vi "plot circles.vi"(2 "dL":dbl=0.5, 3 "Radius":dbl[](array[numeric])=[10.0, 5.0, 8.0, 1.0], 4 "Circle y":dbl[](array[numeric])=[0.0, 3.0, -7.0, -4.0], 5 "Circle x":dbl[](array[numeric])=[0.0, 4.0, -2.0, 2.0]) -> (0 "CY":dbl[](array[numeric]), 1 "CX":dbl[](array[numeric]))   [LabVIEW 2009]
panel:
  out "XY Graph":cluster{dbl[], dbl[]}(graph)
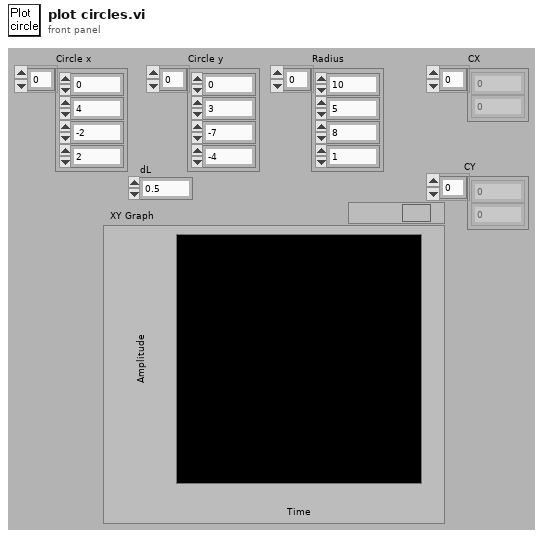
[diagram p1: front panel]
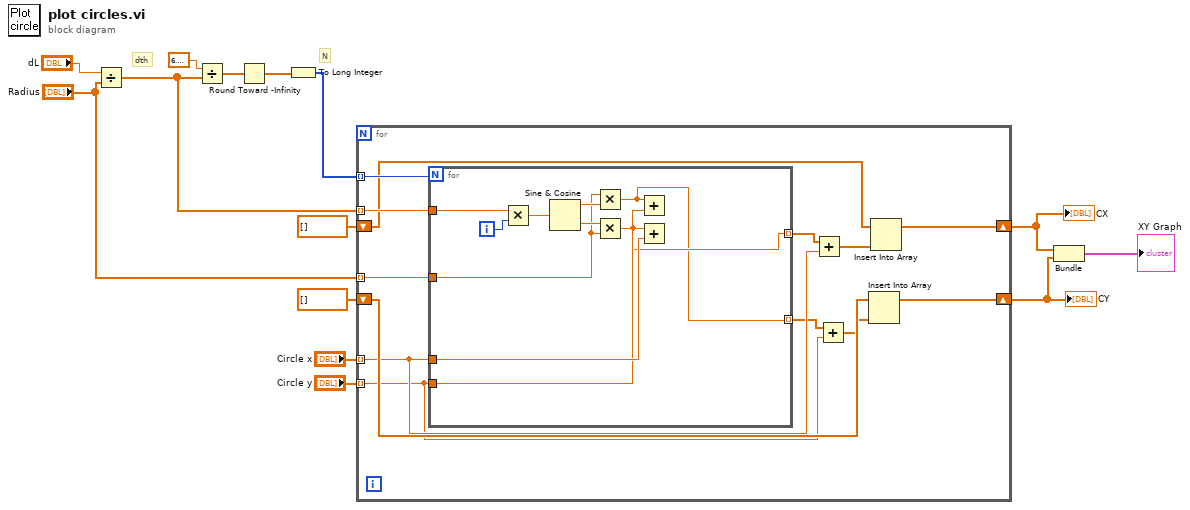
[diagram p0: block diagram]
diagram:
  # "N"
  # "dth"
  n1 = Divide(x="dL", y="Radius") -> (x/y=w9:dbl[])
  n2 = Divide(x=6.283185307179586, y=w9) -> (x/y=w12:dbl[])
  n3 = Round Toward -Infinity(1:w12) -> (0:w11:dbl[])
  n4 = To Long Integer(number=w11) -> (32bit integer=w10:i32[])
  n5 = for {
    tunnel: w10 -> [w27] mode=indexing
    tunnel: w9 -> [w26] mode=indexing
    tunnel: "Circle x" -> [w19] mode=indexing
    tunnel: "Circle y" -> [w16] mode=indexing
    tunnel: "Radius" -> [w25] mode=indexing
    shift-right: [w24] -> w5
    shift-left: dbl[] [] -> [w23]
    shift-right: [w22] -> w4
    shift-left: dbl[] [] -> [w21]
    n6 = for {
      N: w27 -> [_]
      tunnel: w26 -> [w37]
      tunnel: w19 -> [w31]
      tunnel: w16 -> [w30]
      tunnel: w25 -> [w32]
      tunnel: [w28] -> w17 mode=indexing
      tunnel: [w29] -> w20 mode=indexing
      i -> [w36]
      n7 = Multiply(x=w37, y=w36) -> (x*y=w35:dbl)
      n8 = Sine & Cosine(0:w35) -> (1:w33:dbl, 2:w34:dbl)
      n9 = Multiply(x=w32, y=w33) -> (x*y=w28:dbl)
      n10 = Multiply(x=w34, y=w32) -> (x*y=w29:dbl)
      n11 = Add(x=w28, y=w30) -> ()  [unwired: 1 out]
      n12 = Add(x=w29, y=w31) -> ()  [unwired: 1 out]
    }
    n13 = Add(x=w20, y=w19) -> (x+y=w18:dbl[])
    n14 = Add(x=w17, y=w16) -> (x+y=w15:dbl[])
    n15 = Insert Into Array(array=w21, new element=w15) -> (w22:dbl[])  [unwired: 1 in]
    n16 = Insert Into Array(array=w23, new element=w18) -> (w24:dbl[])  [unwired: 1 in]
  }
  "CX" <- w5
  "CY" <- w4
  n17 = Bundle(w5, w4) -> (→"XY Graph":cluster{dbl[], dbl[]})  [unwired: 1 in]
